vi "ftphelp.vi"() -> ()   [LabVIEW 2014]
panel:
  out "Command line arguments for the FTP program that comes with Windows 98 Second Edition (access using >ftp -h).":string="FTP [-v] [-d] [-i] [-n] [-g] [-s:filename] [-a] [-w:windowsize] [-A] [host]\n\n  -v             Suppresses display of remote server responses.\n  -n             Suppresses auto-login upon initial connection.\n  -i             Turns off interactive prompting during multiple file \n                 transfers.\n  -d             Enables debugging.\n  -g             Disables filename globbing (see GLOB command).\n  -s:filename    Specifies a text file containing FTP commands; the \n                 commands will automatically run after FTP starts.\n  -a             Use any local interface when binding data connection.\n  -A             login as anonymous.\n  -w:buffersize  Overrides the default transfer buffer size of 4096.\n  host           Specifies the host name or IP address of the remote\n                 host to connect to."
  out "FTP Commands for the FTP program that comes with Windows 98 Second Edition. (access using ftp> help)":string="!               Escape to the shell\n?               Print local help information\nappend          Append to a file\nascii           Set ascii transfer type\nbell            Beep when command completed\nbinary          Set binary transfer type\nbye             Terminate ftp session and exit\ncd              Change remote working directory\nclose           Terminate ftp session\ndelete          Delete remote file\ndebug           Toggle debugging mode\ndir             List contents of remote directory\ndisconnect      Terminate ftp session\nget             Receive file\nglob            Toggle metacharacter expansion of local file names\nhash            Toggle printing `#' for each buffer transferred\nhelp            Print local help information\nlcd             Change local working directory\nliteral         Send arbitrary ftp command\nls              List contents of remote directory\nmdelete         Delete multiple files\nmdir            List contents of multiple remote directories\nmget            Get multiple files\nmkdir           Make directory on the remote machine\nmls             List contents of multiple remote directories\nmput            Send multiple files\nopen            Connect to remote tftp\nprompt          Force interactive prompting on multiple commands\nput             Send one file\npwd             Print working directory on remote machine\nquit            Terminate ftp session and exit\nquote           Send arbitrary ftp command\nrecv            Receive file\nremotehelp      Get help from remote server\nrename          Rename file\nrmdir           Remove directory on the remote machine\nsend            Send one file\nstatus          Show current status\ntrace           Toggle packet tracing\ntype            Set file transfer type\nuser            Send new user information\nverbose         Toggle verbose mode"
  out "Remote FTP commands for the RT Engine's FTP Server (access using ftp>remotehelp)":string="ABOR Abort previous FTP service command\nACCT Argument identifies the user's account (unimplemented)\nALLO Reserve storage\nAPPE Append to file\nCDUP Change to parent directory\nCWD  Change working directory\nDELE Delete file\nHELP Send helpful information\nLIST Send file list\nMKD  Create a directory\nMODE Specify the transfer mode (only STREAM implemented)\nNLST Send a list of file names\nNOOP No operation\nPASS Argument is the user's password\nPASV Cause the server to listen on the data port\nPORT Data port to be used in data connection\nPWD  Print working directory\nQUIT Terminate service\nREIN Reinitialize control connection (unimplemented)\nREST Restart transfer (unimplemented)\nRETR Retrieve file\nRMD  Remove directory\nRNFR Rename from\nRNTO Rename to\nSITE System specific services: FNS protection=mask owner=name group=name\nSIZE Get the size of a file\nSMNT Structure mount (unimplemented)\nSTAT Status information\nSTOR Store file\nSTOU Store unique file\nSTRU File structure (only FILE implemented)\nSYST System type\nTYPE Representation type (EBCDIC unimplemented)\nUSER User \nXCUP Change to parent directory\nXMKD Create a directory\nXPWD Print working directory\nXRMD Remove directory"
  in  "OK Button":bool
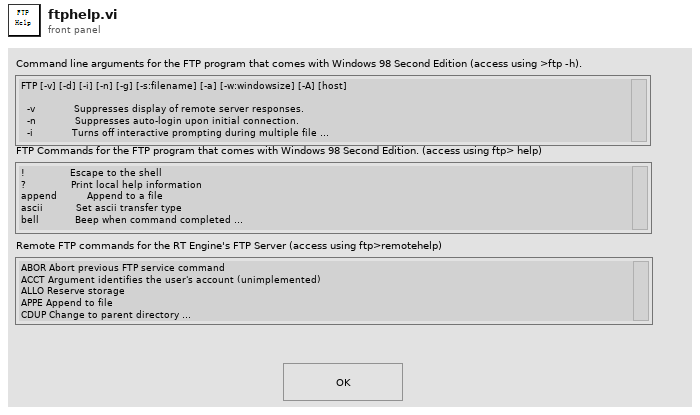
[diagram p1: front panel]
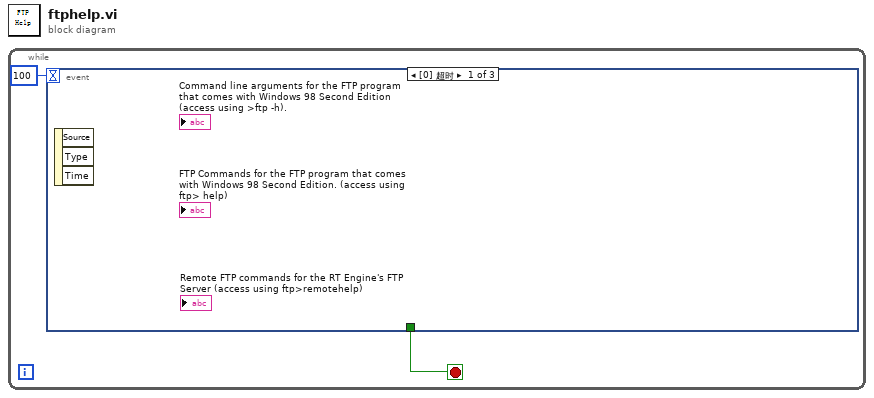
[diagram p0: block diagram]
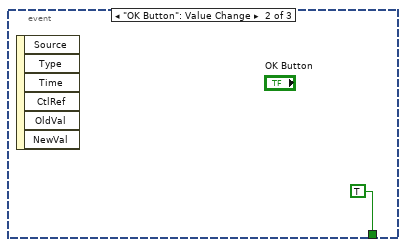
[diagram p2: hidden frame]
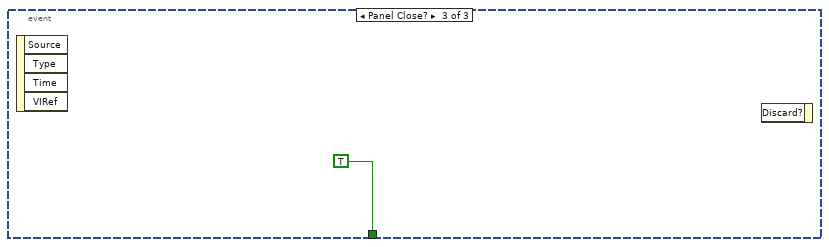
[diagram p3: hidden frame]
diagram:
  n1 = while {
    stop <- w2 stop-if-true
    n2 = event shown="[0] 超时" {
      selector: _ -> [_ _ _]
      dyn-events: _ -> [_ _ _]
      timeout: 100 -> [_ _ _]
      tunnel: [_ TRUE TRUE] -> w2
      event Timeout {
        n3 = event-data() -> ()  [unwired: 1 in, 3 out]
      }
      event "OK Button": Value Change {
        n4 = event-data() -> ()  [unwired: 1 in, 6 out]
      }
      event Panel Close? {
        n5 = event-data() -> ()  [unwired: 1 in, 4 out]
        n6 = event-data() -> ()  [unwired: 2 in, 1 out]
      }
    }
  }
